vi "CreateBotSpeak.vi"() -> (3 "VIA out":refnum<class "BotSpeak.lvclass">)   [LabVIEW 2012, in "BotSpeakManager.lvclass"]
uses:
  <vilib>/NXT/LegoClasses/BrickManagers/BotSpeakManager/BotSpeakManager.lvclass
  <userlib>/botspeak/VIs/BotSpeak.lvclass
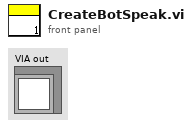
[diagram p1: front panel]
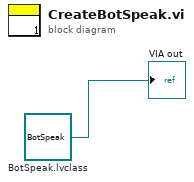
[diagram p0: block diagram]
diagram:
  w1 = refnum<class "BotSpeak.lvclass"> refnum  # BotSpeak.lvclass
  "VIA out" <- w1
